vi "CommandSelect.vi"(9 "Config Sel":bool, 10 "A/D Settings":u16(ring) items=["512", "2048", "Set to HF 1080", "Capacitance on CH0", "Request dividers", "Set to LF 356", "Enable CH0 only", "Enable CH1 only", "Pause", "Single sample"], 11 "Command":u16(ring) items=["Read 256 bytes", "Read Both Channels 2048 b", "Request Dividers", "Enable CH0 only", "Enable CH1 only", "Pause", "Single sample"]) -> (3 "Command Out":string)   [LabVIEW 2012]
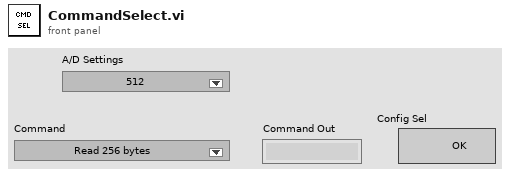
[diagram p1: front panel]
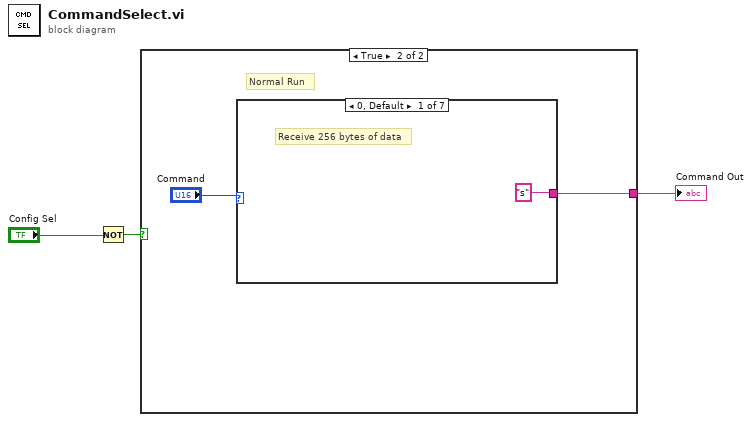
[diagram p0: block diagram]
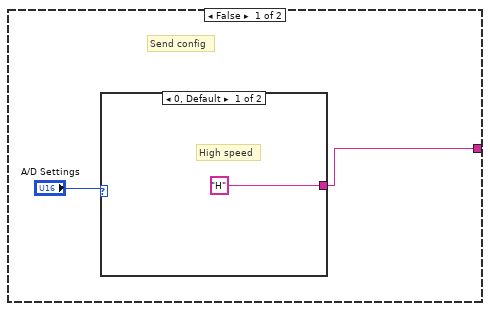
[diagram p2: hidden frame]
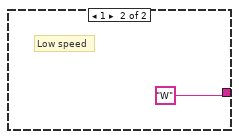
[diagram p3: hidden frame]
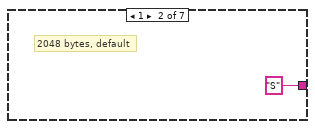
[diagram p4: hidden frame]
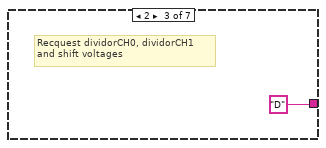
[diagram p5: hidden frame]
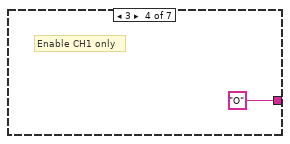
[diagram p6: hidden frame]
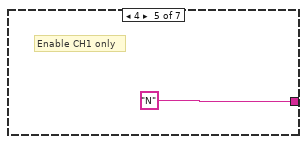
[diagram p7: hidden frame]
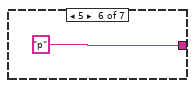
[diagram p8: hidden frame]
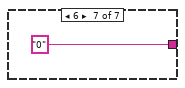
[diagram p9: hidden frame]
diagram:
  n1 = Not(x="Config Sel") -> (.not. x?=w3:bool)
  n2 = case shown="True" w3 {
    tunnel: [w5 w8] -> w1
    frame False {
      # "Send config"
      n3 = case shown="0, Default" "A/D Settings" {
        tunnel: ["H" "W"] -> w5
        frame 0, Default {
          # "High speed"
        }
        frame 1 {
          # "Low speed"
        }
      }
    }
    frame True {
      # "Normal Run"
      n4 = case shown="0, Default" "Command" {
        tunnel: ["s" "S" "D" "O" "N" "p" "0"] -> w8
        frame 0, Default {
          # "Receive 256 bytes of data"
        }
        frame 1 {
          # "2048 bytes, default"
        }
        frame 2 {
          # "Recquest dividorCH0, dividorCH1\nand shift voltages"
        }
        frame 3 {
          # "Enable CH1 only"
        }
        frame 4 {
          # "Enable CH1 only"
        }
        frame 5 {
        }
        frame 6 {
        }
      }
    }
  }
  "Command Out" <- w1
